vi "AlazarCoprocessorRegisterRead.vi"(0 "Handle":u64, 1 "Offset":u32, 2 "error in (no error)":errorcluster) -> (3 "Handle":u64, 4 "Value":u32, 5 "Return Code":u32, 6 "error out":errorcluster)   [LabVIEW 2009]
doc: "Read the contents of a user-programmable coprocessor FPGA register."
uses:
  ATSApi.dll
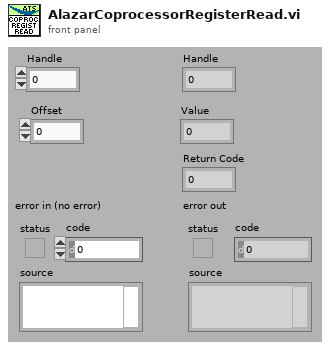
[diagram p1: front panel]
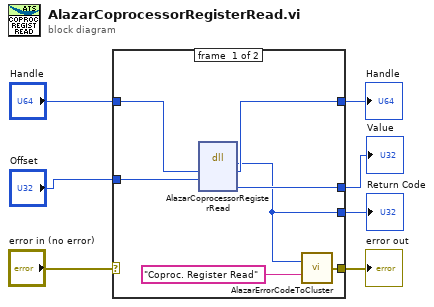
[diagram p0: block diagram]
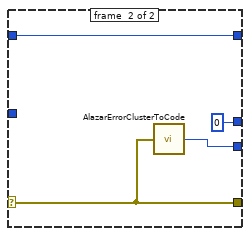
[diagram p2: hidden frame]
diagram:
  n1 = case shown="No Error" "error in (no error)" {
    selector: "error in (no error)" -> [_ w18]
    tunnel: [w10 w18] -> w6
    tunnel: [w9 w17] -> w5
    tunnel: "Handle" -> [w14 w16]
    tunnel: [w13 w16] -> w3
    tunnel: [w12 u32 0] -> w2
    tunnel: "Offset" -> [w11 _]
    frame #0 {
      n2 = dll-call lib="ATSApi.dll" fn="AlazarCoprocessorRegisterRead"("handle"=w14, "offset"=w11) -> ("return type"=w9:u32, "handle"=w13:u64, "value"=w12:u32)  [unwired: 5 in, 2 out]
      n3 = call "AlazarErrorCodeToCluster.vi"("Message"="Coproc. Register Read", "Error Code"=w9) -> ("error out"=w10:errorcluster)
    }
    frame #1 {
      n4 = call "AlazarErrorClusterToCode.vi"("error in (no error)"=w18) -> ("Error Code"=w17:u32)
    }
  }
  "Handle" <- w3
  "error out" <- w6
  "Return Code" <- w5
  "Value" <- w2
